vi "Read Piezo Voltage.vi"(0 "object in":refnum<class "TBS2000Series.lvclass">, 5 "error in (no error)":errorcluster) -> (14 "object out":refnum<class "TBS2000Series.lvclass">, 15 "Peak-to-Peak":dbl format="%.2p", 16 "Frequency":dbl format="%.2p", 17 "Piezo Voltage Prefocus Channel":T1(graph), 19 "error out":errorcluster)   [LabVIEW 2023, in "TBS2000Series.lvclass"]
uses:
  TBS2000Series.lvclass
  TBS2000Series.lvclass/TBS2000Series.ctl
  <instrlib>/Tektronix TBS 2000 Series/Tektronix TBS 2000 Series.lvlib
panel:
  in  "Timebase (4.00 us)":dbl=4e-06 format="%.2p"
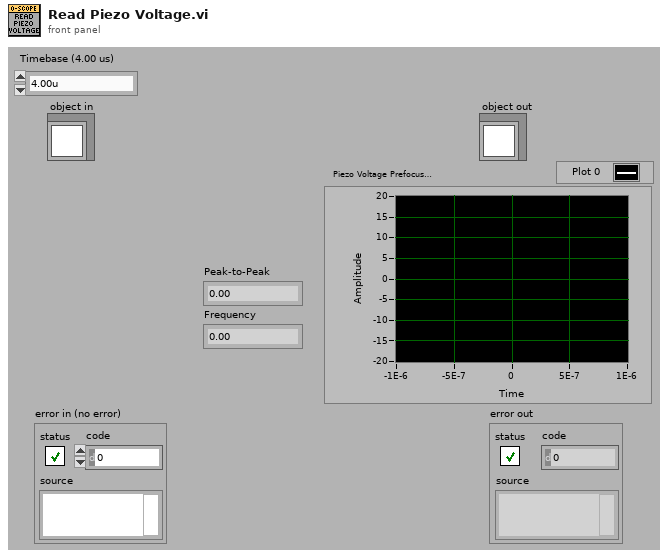
[diagram p1: front panel]
types:
  T1 = cluster{"Initial X":dbl, "X Increment":dbl, "Waveform Array":dbl[]}
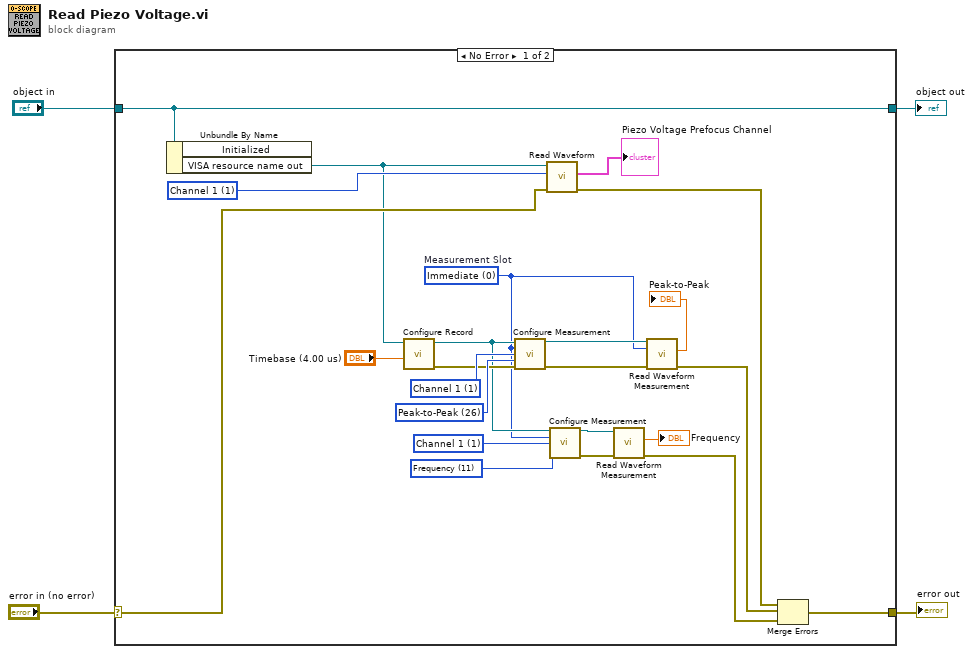
[diagram p0: block diagram]
diagram:
  n1 = case shown="No Error" "error in (no error)" {
    selector: "error in (no error)" -> [w19 w29]
    tunnel: [w18 w29] -> w3
    tunnel: [w27 w28] -> w1
    tunnel: "object in" -> [w27 w28]
    frame No Error {
      w14 = 11 items=["Amplitude", "Area", "Burst", "Cycle Area", "Cycle Mean", "Cycle RMS", "Delay RR", "Delay RF", "Delay FR", "Delay FF", "Fall Time", "Frequency", "High Reference", "Low Reference", "Max", "Mean", "Min", "- Duty Cycle", "- Edge Count", "- Overshoot", "- Pulse Count", "- Width", "+ Duty Cycle", "+ Edge Count", "Period", "Phase", "Peak-to-Peak", "+ Overshoot", "+ Pulse Count", "+ Width", "Rise", "RMS"] ("Measurement Type (30: Rise)")
      w15 = 1 items=["Math", "Channel 1", "Channel 2", "Channel 3", "Channel 4"] ("Measurement Source 1 (1: Channel 1)")
      w23 = 26 items=["Amplitude", "Area", "Burst", "Cycle Area", "Cycle Mean", "Cycle RMS", "Delay RR", "Delay RF", "Delay FR", "Delay FF", "Fall Time", "Frequency", "High Reference", "Low Reference", "Max", "Mean", "Min", "- Duty Cycle", "- Edge Count", "- Overshoot", "- Pulse Count", "- Width", "+ Duty Cycle", "+ Edge Count", "Period", "Phase", "Peak-to-Peak", "+ Overshoot", "+ Pulse Count", "+ Width", "Rise", "RMS"] ("Measurement Type (0: Amplitude)")
      w22 = 1 items=["Math", "Channel 1", "Channel 2", "Channel 3", "Channel 4"] ("Measurement Source 1 (1: Channel 1)")
      w8 = 0 items=["Immediate", "Measurement 1", "Measurement 2", "Measurement 3", "Measurement 4", "Measurement 5", "Measurement 6"]  # Measurement Slot
      w26 = 1 items=["Math", "Channel 1", "Channel 2", "Channel 3", "Channel 4"] ("Source (1: Channel 1)")
      n2 = Unbundle By Name(w27) -> ("VISA resource name out"=w16:refnum<visa-resource-name>)  [unwired: 1 out]
      n3 = call <instrlib>:"Configure Record.vi"("Timebase (4.00 us)"="Timebase (4.00 us)", "VISA resource name"=w16) -> ("error out"=w21:errorcluster, "VISA resource name out"=w9:refnum<visa-resource-name>)  [unwired: 8 in]
      n4 = call <instrlib>:"Configure Measurement.vi"("VISA resource name"=w9, "Measurement Slot (0: Immediate)"=w8, "Measurement Source 1 (1: Channel 1)"=w22, "Measurement Type (30: Rise)"=w23, "error in (no error)"=w21) -> ("VISA resource name out"=w13:refnum<visa-resource-name>, "error out"=w12:errorcluster)  [unwired: 9 in]
      n5 = call <instrlib>:"Read Waveform.vi"("error in (no error)"=w19, "Source (1: Channel 1)"=w26, "VISA resource name"=w16) -> ("error out"=w17:errorcluster, "Waveform Graph"=→"Piezo Voltage Prefocus Channel":T1)  [unwired: 6 in, 1 out]
      n6 = call <instrlib>:"Configure Measurement.vi"("VISA resource name"=w9, "Measurement Slot (0: Immediate)"=w8, "Measurement Source 1 (1: Channel 1)"=w15, "Measurement Type (30: Rise)"=w14) -> ("VISA resource name out"=w11:refnum<visa-resource-name>, "error out"=w10:errorcluster)  [unwired: 10 in]
      n7 = call <instrlib>:"Read Waveform Measurement.vi"("error in (no error)"=w10, "VISA resource name"=w11) -> ("error out"=w5:errorcluster, "Measurement"=→"Frequency":dbl)  [unwired: 7 in, 1 out]
      n8 = call <instrlib>:"Read Waveform Measurement.vi"("error in (no error)"=w12, "Measurement Slot (0: Immediate)"=w8, "VISA resource name"=w13) -> ("error out"=w6:errorcluster, "Measurement"=→"Peak-to-Peak":dbl)  [unwired: 6 in, 1 out]
      n9 = Merge Errors(w17, w6, w5) -> (w18:errorcluster)
    }
    frame Error {
    }
  }
  "error out" <- w3
  "object out" <- w1
